vi "OpenFP_CreateUE.vi"(0 "VI_Reference_In":refnum<vi>, 5 "Exec.State":T1(ring), 11 "Error_In":errorcluster) -> (4 "VI_Reference_Out":refnum<vi>, 15 "Error_Out":errorcluster)   [LabVIEW 2023]
doc: "Used to open the Front panel and Create the User Event"
uses:
  Controls/Open_Close.ctl
  Controls/Operation.ctl
  Controls/Event_Data.ctl
  LV2/UE_C_LV2.vi
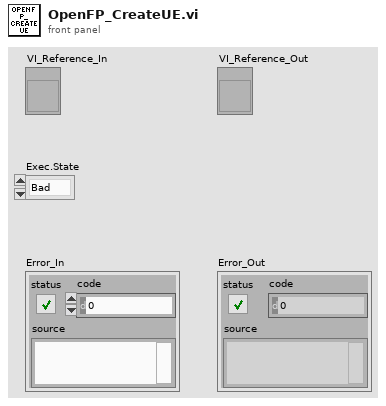
[diagram p1: front panel]
types:
  T1 = enum32{"Bad", "Idle", "Run top level", "Running"}
  T2 = typedef "Event_Data.ctl" = cluster{"Event_Data":dbl, "PlayBack?":bool}
  T3 = typedef "Operation.ctl" = enum16{"Create_UE", "Generate_UE", "Destroy_UE", "Get_UE_Reference"}
  T4 = typedef "Open_Close.ctl" = enum16{"Open", "Close"}
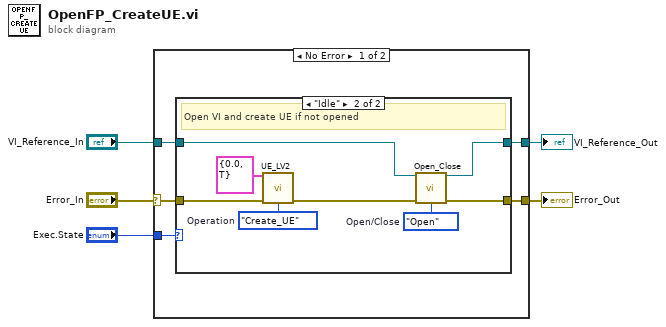
[diagram p0: block diagram]
diagram:
  n1 = case shown="No Error" "Error_In" {
    selector: "Error_In" -> [w6 w22]
    tunnel: [w10 w22] -> w5
    tunnel: "VI_Reference_In" -> [w9 w21]
    tunnel: "Exec.State" -> [w8 _]
    tunnel: [w7 w21] -> w2
    frame No Error {
      n2 = case shown="\"Idle\"" w8 {
        tunnel: [w12 w20] -> w10
        tunnel: w6 -> [w12 w13]
        tunnel: w9 -> [w11 w14]
        tunnel: [w11 w18] -> w7
        frame "Bad", Default {
        }
        frame "Idle" {
          w16 = Operation."Create_UE"  # Operation
          w19 = Open_Close."Open"  # Open/Close
          # "Open VI and create UE if not opened"
          n3 = call-poly "UE_LV2.vi"("Event_Data"=T2 {"Event_Data"=0.0, "PlayBack?"=TRUE}, "Error_In"=w13, "Operation"=w16) -> ("Error_Out"=w17:errorcluster)  [unwired: 11 in, 1 out]
          n4 = call "Open_Close.vi"("VI_Reference_In"=w14, "Error_In"=w17, "Open/Close"=w19) -> ("VI_Reference_Out"=w18:refnum<vi>, "Error_Out"=w20:errorcluster)  [unwired: 11 in]
        }
      }
    }
    frame Error {
    }
  }
  "Error_Out" <- w5
  "VI_Reference_Out" <- w2
